vi "Setup Test.vi"(4 "error in":errorcluster) -> (0 "error out":errorcluster)   [LabVIEW 2025]
doc: "This VI prepares Unit testing of the project. It creates VIs and Projects according to the specification files."
uses:
  <userlib>/_OpenG.lib/file/file.llb/openg_file.lvlib
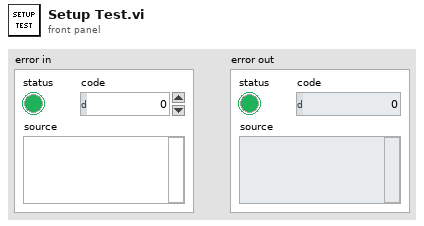
[diagram p1: front panel]
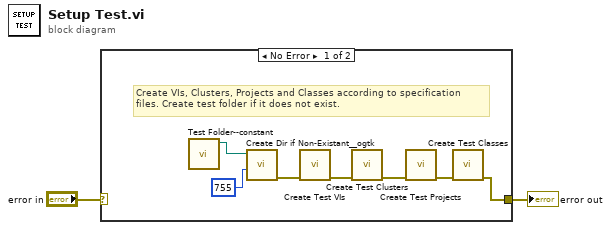
[diagram p0: block diagram]
diagram:
  n1 = case shown="No Error" "error in" {
    selector: "error in" -> [_ w10]
    tunnel: [w5 w10] -> w1
    frame No Error {
      # "Create VIs, Clusters, Projects and Classes according to specification\nfiles. Create test folder if it does not exist."
      n2 = call "Test Folder--constant.vi"() -> ("Test Folder"=w7:path)  [unwired: 7 in]
      n3 = call <userlib>:"Create Dir if Non-Existant__ogtk.vi"("permissions (0755)"=i16 755, "Directory Path"=w7) -> ("error out"=w9:errorcluster)  [unwired: 7 in, 2 out]
      n4 = call "Create Test VIs.vi"("error in"=w9) -> ("error out"=w4:errorcluster)  [unwired: 6 in]
      n5 = call "Create Test Clusters.vi"("error in"=w4) -> ("error out"=w3:errorcluster)  [unwired: 6 in]
      n6 = call "Create Test Projects.vi"("error in"=w3) -> ("error out"=w6:errorcluster)  [unwired: 6 in]
      n7 = call "Create Test Classes.vi"("error in"=w6) -> ("error out"=w5:errorcluster)  [unwired: 6 in]
    }
    frame Error {
      # "Pass error without further action"
    }
  }
  "error out" <- w1
